vi "Create Mock Single Input.vi"(7 "VI Name":string, 8 "error in (no error)":errorcluster, 9 "Control value":variant, 10 "Control Label":string) -> (0 "error out":errorcluster, 3 "Mock VI Call Out":refnum<class "Mock VI Call.lvclass">)   [LabVIEW 2020, in "Mock VI Call.lvclass"]
uses:
  Mock VI Call.lvclass
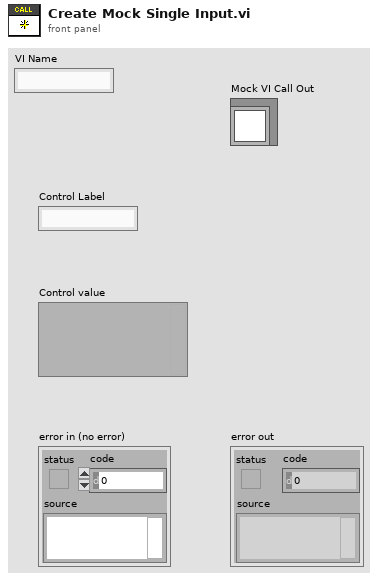
[diagram p1: front panel]
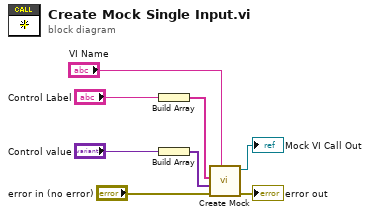
[diagram p0: block diagram]
diagram:
  n1 = Build Array("Control Label") -> (w4:string[])
  n2 = Build Array("Control value") -> (w5:variant[])
  n3 = call "Create Mock.vi"("VI Name"="VI Name", "error in (no error)"="error in (no error)", "Control value"=w5, "Control Label"=w4) -> ("error out"=→"error out":errorcluster, "Mock VI Call Out"=→"Mock VI Call Out":refnum<class "Mock VI Call.lvclass">)  [unwired: 6 in]
